vi "Send stream_TTTR.vi"(0 "Message Enqueuer":refnum<class "Message Enqueuer.lvclass">, 1 "Message Priority (Normal)":T6=enum."Normal", 2 "Log Type":T1, 5 "fifo_stream_path":path, 7 "Correlation_settings":T2 {"Lag Settings"."time_start" items=["1 ps"=1, "10 ps"=10, "100 ps"=100, "1 ns"=1000, "10 ns"=10000, "100 ns"=100000, "1 us"=1000000, "10 us"=10000000, "100 us"=100000000, "1 ms"=1000000000, "10 ms"=10000000000, "100 ms"=100000000000, "1 s"=1000000000000, "10 s"=10000000000000, "100 s"=100000000000000]; "Lag Settings"."time_end" items=["1 ps"=1, "10 ps"=10, "100 ps"=100, "1 ns"=1000, "10 ns"=10000, "100 ns"=100000, "1 us"=1000000, "10 us"=10000000, "100 us"=100000000, "1 ms"=1000000000, "10 ms"=10000000000, "100 ms"=100000000000, "1 s"=1000000000000, "10 s"=10000000000000, "100 s"=100000000000000]}, 9 "action_for_records":T5, 11 "error in (no error)":errorcluster, 12 "acq_time":i32, 13 "Stream Notes":string, 14 "stop_fifo_stream":refnum<event-registration>) -> (4 "Message Enqueuer out":refnum<class "Message Enqueuer.lvclass">, 15 "error out":errorcluster)   [LabVIEW 2015, in "stream_TTTR Msg.lvclass"]
doc: "This VI sends the message to an actor."
uses:
  stream_TTTR Msg.lvclass
  <vilib>/ActorFramework/Message Enqueuer/Message Enqueuer.lvclass
  <vilib>/ActorFramework/Message Enqueuer/Message Priority.ctl
  hydraharp/hydraharp_action_on_records.ctl
  hydraharp_panel/hpanel_correlation_settings.ctl
  hydraharp/hydraharp_correlation_lag_settings.ctl
  hydraharp/hydraharp_time_decades.ctl
  record_type.ctl
  stream_TTTR Msg.lvclass/stream_TTTR Msg.ctl
  <vilib>/ActorFramework/Message Enqueuer/Message Enqueuer.lvclass/Message Enqueuer.ctl
  <vilib>/ActorFramework/Message Priority Queue/Priority Enqueue.vi
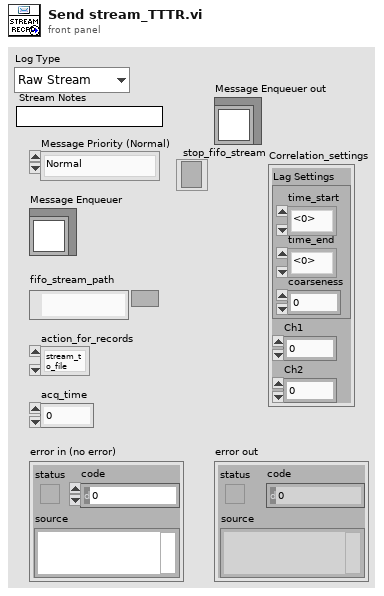
[diagram p1: front panel]
types:
  T1 = typedef "record_type.ctl" = enum16{"Raw Stream", "Processed Records (hdf5)"}
  T2 = typedef "hpanel_correlation_settings.ctl" = cluster{"Lag Settings":T3, "Ch1":u8, "Ch2":u8}
  T3 = typedef "hydraharp_correlation_lag_settings.ctl" = cluster{"time_start":T4, "time_end":T4, "coarseness":i64}
  T4 = typedef "hydraharp_time_decades.ctl" = i64
  T5 = typedef "hydraharp_action_on_records.ctl" = enum16{"stream_to_file", "correlate", "stream to file and correlate", "histogram"}
  T6 = typedef "Actor Framework.lvlib/Message Enqueuer.lvclass/Message Priority.ctl" = enum16{"Low", "Normal", "High"}
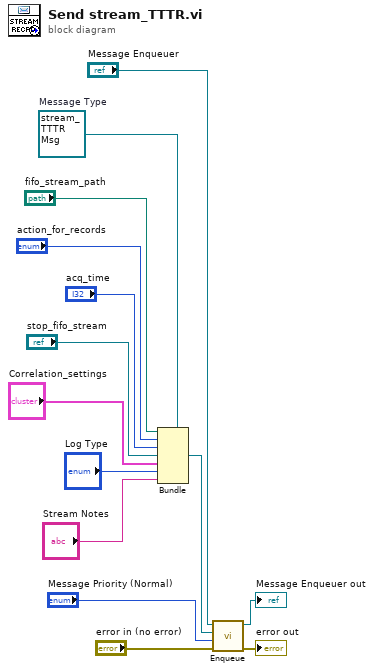
[diagram p0: block diagram]
diagram:
  w11 = refnum<class "stream_TTTR Msg.lvclass"> refnum  # Message Type
  n1 = Bundle(cluster=w11, "fifo_stream_path", "action_for_records", "acq_time", "stop_fifo_stream", "Correlation_settings", "Log Type", "Stream Notes") -> (w10:refnum<class "stream_TTTR Msg.lvclass">)
  n2 = call <vilib>:"Enqueue.vi"("error in (no error)"="error in (no error)", "Message Priority (Normal)"="Message Priority (Normal)", "Message"=w10, "Message Enqueuer in"="Message Enqueuer") -> ("error out"=→"error out":errorcluster, "Message Enqueuer out"=→"Message Enqueuer out":refnum<class "Message Enqueuer.lvclass">)  [unwired: 6 in]
